vi "FTW-Connector-SpawnNewActor-Strict.vi"(0 "FTW Actor Connector Type":refnum<class "FTW-ActorConnector.lvclass">, 1 "Configuration":string="{}", 5 "Identity":string, 7 "Actor VI Filepath":path, 9 "Timeout":i32=-2 format="%dmsec", 11 "error in":errorcluster) -> (4 "FTW Actor Connector":refnum<class "FTW-ActorConnector.lvclass">, 6 "Initialized Response":string, 8 "Instance Inbox Address":string, 15 "error out":errorcluster)   [LabVIEW 2015, in "FTW-ActorConnector.lvclass"]
doc: "Spawn a new actor with the minimum required parameters"
uses:
  FTW-ActorConnector.lvclass
panel:
  # "Inputs"
  # "Outputs"
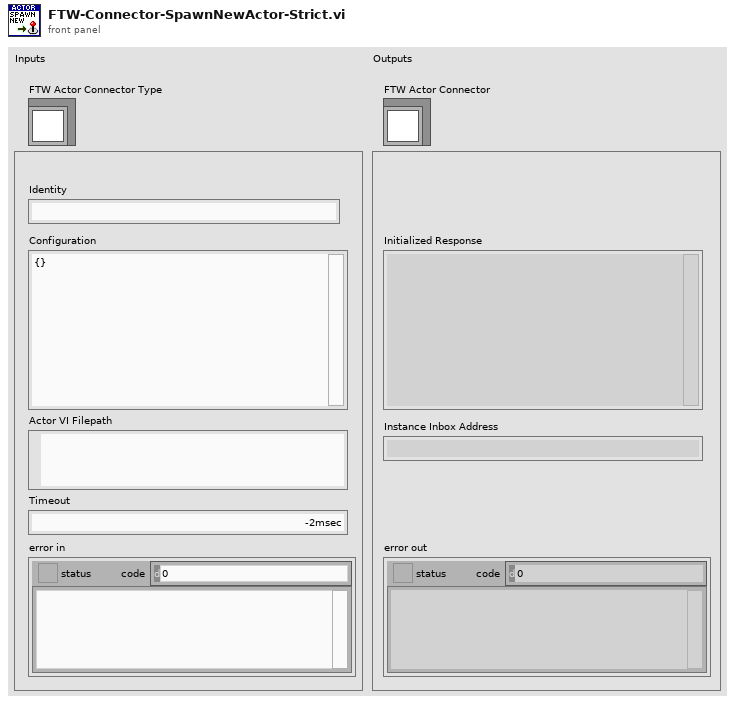
[diagram p1: front panel]
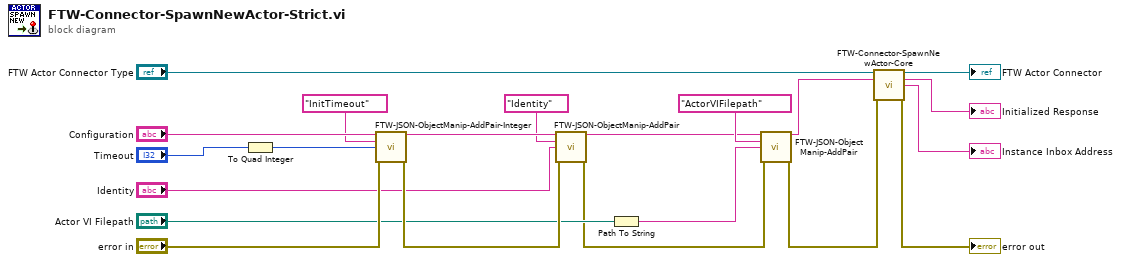
[diagram p0: block diagram]
diagram:
  n1 = To Quad Integer(1:"Timeout") -> (0:w12:i64)
  n2 = call "FTW-JSON-ObjectManip-AddPair-Integer.vi"("Input JSON Object"="Configuration", "Key"="InitTimeout", "Value"=w12, "error in"="error in") -> ("Output JSON Object"=w5:string, "error out"=w10:errorcluster)  [unwired: 10 in]
  n3 = call "FTW-JSON-ObjectManip-AddPair.vi"("Input JSON Object"=w5, "Key"="Identity", "Value"="Identity", "error in"=w10) -> ("Output JSON Object"=w4:string, "error out"=w6:errorcluster)  [unwired: 10 in]
  n4 = Path To String(path="Actor VI Filepath") -> (string=w1:string)
  n5 = call "FTW-JSON-ObjectManip-AddPair.vi"("Input JSON Object"=w4, "Key"="ActorVIFilepath", "Value"=w1, "error in"=w6) -> ("Output JSON Object"=w11:string, "error out"=w9:errorcluster)  [unwired: 10 in]
  n6 = call "FTW-Connector-SpawnNewActor-Core.vi"("FTW Actor Connector Type"="FTW Actor Connector Type", "Configuration"=w11, "error in"=w9) -> ("FTW Actor Connector"=→"FTW Actor Connector":refnum<class "FTW-ActorConnector.lvclass">, "Initialized Response"=→"Initialized Response":string, "Instance Inbox Address"=→"Instance Inbox Address":string, "error out"=→"error out":errorcluster)  [unwired: 9 in]
